vi "MSC ROI to IMAQ ROI.vi"(0 "ROIs":T1[](array[typedef]) {"Type" items=["Point", "Line", "Rectangle", "Oval", "Freehand / Polygon"]}, 11 "error in":errorcluster) -> (4 "IMAQ ROI Descriptor":T5 {"Contours"."Type" items=["No Selection", "Point", "Line", "Rectangle", "Oval", "Polygon", "Freehand Region", "Annulus", "Unused2", "Unused3", "Broken Line", "Freehand Line", "Rotated Rectangle"]}, 15 "error out":errorcluster)   [LabVIEW 2014]
doc: "Converts MSC ROIs to an IMAQ ROI Descriptor\n\n<B>Currently supported:</B>\n- Point\n- Line\n- Rectangle\n- Oval\n- Polygon\n- Freehand Region"
uses:
  MSC Image_class/controls/ROI.ctl
  MSC Image_class/controls/ROI Type.ctl
  MSC Image_class/controls/Contour.ctl
  MSC Image_class/controls/Contour hierarchy.ctl
  MSC Image_class/MSC Image.lvclass
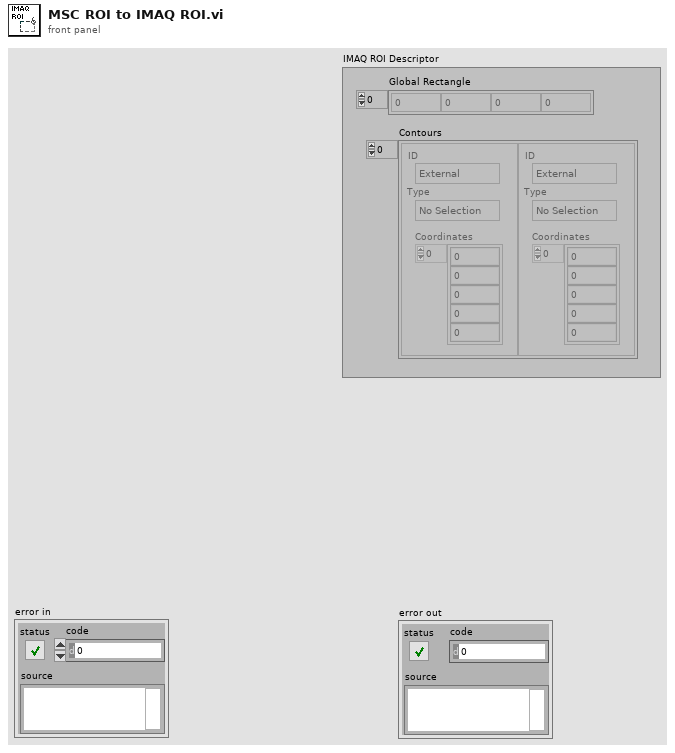
[diagram p1: front panel]
types:
  T1 = typedef "MSC Image.lvclass/ROI.ctl" = cluster{"Type":T2, "Parameters":dbl[], "Contour":T3, "Bounding Box":T3, "Contour Length":dbl, "ROI Area":dbl, "ROI Mean":dbl, "ROI Standard Deviation":dbl, "ROI Min":dbl, "ROI Max":dbl, "Hierarchy":T4, "Variant":variant, "Timestamp":timestamp}
  T2 = typedef "MSC Image.lvclass/ROI Type.ctl" = u16
  T3 = typedef "MSC Image.lvclass/Contour.ctl" = cluster{"x":i16, "y":i16}[]
  T4 = typedef "MSC Image.lvclass/Contour hierarchy.ctl" = cluster{"parent ID":i32, "children IDs":dbl[], "level":i32}
  T5 = typedef "ROI Descriptor" = cluster{"Global Rectangle":i32[], "Contours":cluster{"ID":enum32{"External", "Internal"}, "Type":u32, "Coordinates":i32[]}[]}
  T6 = cluster{"ID":enum32{"External", "Internal"}, "Type":u32, "Coordinates":i32[]}
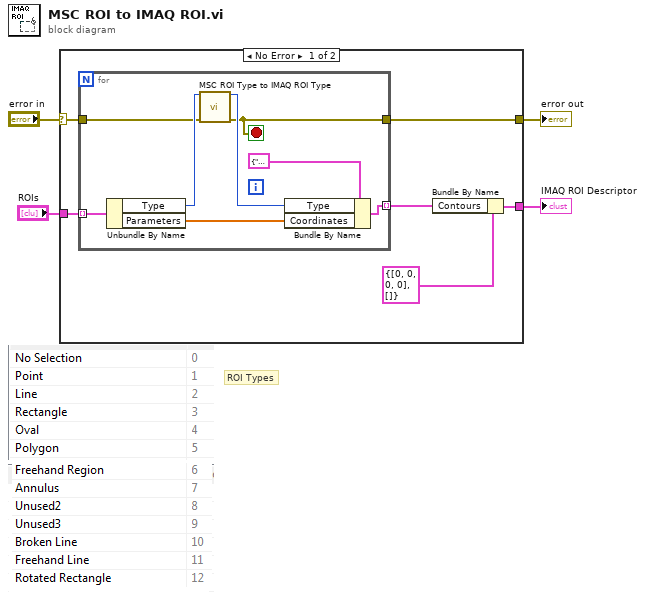
[diagram p0: block diagram]
diagram:
  # "ROI Types"
  n1 = case shown="No Error" "error in" {
    selector: "error in" -> [w9 w19]
    tunnel: [w10 w19] -> w4
    tunnel: "ROIs" -> [w8 _]
    tunnel: [w5 _] -> w1
    frame No Error {
      n2 = for {
        tunnel: w9 -> [w13]
        tunnel: [w12] -> w10
        tunnel: w8 -> [w18] mode=indexing
        tunnel: [w11] -> w6 mode=indexing
        stop <- w12 stop-if-true
        n3 = Unbundle By Name(w18) -> ("Type"=w16:T2, "Parameters"=w14:dbl[])
        n4 = call "MSC ROI Type to IMAQ ROI Type.vi"("MSC ROI Type"=w16, "error in (no error)"=w13) -> ("IMAQ ROI Type"=w15:u32, "error out"=w12:errorcluster)  [unwired: 12 in]
        n5 = Bundle By Name(cluster=T6 {"ID"=enum."External", "Type"=0, "Coordinates"=[]}, "Type"=w15, "Coordinates"=w14) -> (w11:T6)
      }
      n6 = Bundle By Name(cluster=T5 {"Global Rectangle"=[0, 0, 0, 0], "Contours"=[]} ("IMAQ ROI Descriptor"), "Contours"=w6) -> (w5:T5)
    }
    frame Error {
    }
  }
  "IMAQ ROI Descriptor" <- w1
  "error out" <- w4
